vi "io-find-by-address.vi"(10 "Device Address":u8, 11 "UiIoConfig":T1[](array[typedef]) {"calibration"."Y" format="%#.3f"; "calibration"."X" format="%#.3f"; "ADDR" format="%04d"}) -> (3 "Array":T1[](array[typedef]) {"calibration"."Y" format="%#.3f"; "calibration"."X" format="%#.3f"; "ADDR" format="%04d"})   [LabVIEW 2024]
uses:
  controls/IONode.ctl
  controls/type.address.ctl
  controls/enum.io.type.ctl
  controls/enum.io.mode.ctl
  controls/typeXyPoint.ctl
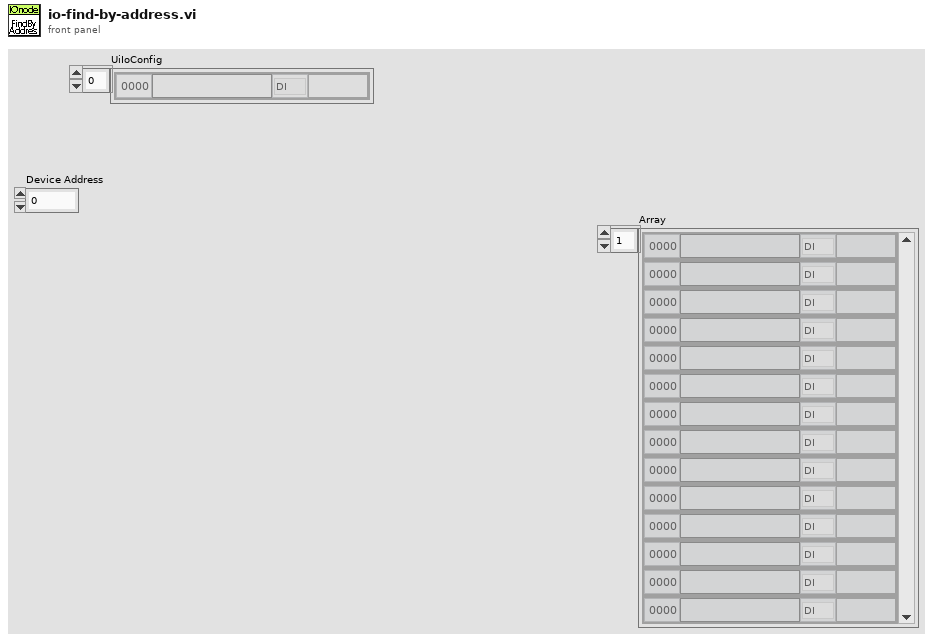
[diagram p1: front panel]
types:
  T1 = typedef "IONode.ctl" = cluster{"ADDR":T2, "Label":string, "Type":T3, "Mode":T4, "Value":string, "Tags":string, "calibration":T5[]}
  T2 = typedef "type.address.ctl" = u16
  T3 = typedef "enum.io.type.ctl" = enum16{"Type", "DI", "DO", "AI", "AO", "VL", "BUF"}
  T4 = typedef "enum.io.mode.ctl" = enum16{"Mode", "RIO", "SIM"}
  T5 = typedef "typeXyPoint.ctl" = cluster{"X":dbl, "Y":dbl}
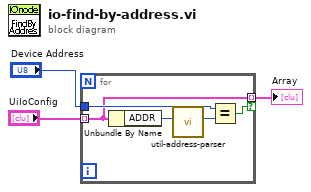
[diagram p0: block diagram]
diagram:
  n1 = for {
    tunnel: "UiIoConfig" -> [w7] mode=indexing
    tunnel: "Device Address" -> [w8]
    tunnel: [w7] -> w3 mode=indexing if=w6
    n2 = Unbundle By Name(w7) -> ("ADDR"=w5:T2)
    n3 = call "util-address-parser.vi"("ADDR 2"=w5) -> ("Address"=w4:u8)  [unwired: 9 in, 1 out]
    n4 = Equal?(x=w8, y=w4) -> (x = y?=w6:bool)
  }
  "Array" <- w3
